vi "Message Console.vi"(7 "Name":string="MessageConsole") -> ()   [LabVIEW 2017, in "DebugConsole.lvlib"]
doc: "CSM Debug Console, you can use this tool:\n\n1. Select an existing CSM instance, open the front panel and block diagram.\n2. Scan the API interfaces of existing CSM instances.\n3. Select an API interface, call synchronously or asynchronously, view the return value.\n4. View the overall program's running log."
uses:
  DebugConsole.lvlib
  _Support/GlobalEvent/LogFilter/LogFilter.lvclass/LogFilter.ctl
  _Support/Typedef/_CSM_GlobalLog_MSG.ctl
  _Support/Typedef/_CSM_Response Source Message.ctl
  _Support/Typedef/_CSM_GlobalLog_MSG_TYPE.ctl
  _Support/Typedef/_CSM_List Module Scope.ctl
  _BroadcastDef.ctl
  _Polymophic/Build Synchronous Message with Arguments.vi
  _Polymophic/Build No-Reply Asynchronous Message with Arguments.vi
  _Polymophic/Build Interrupt Broadcast Message.vi
  AdvanceAPI/CSM - Convert Error to Argument.vi
  _Support/GlobalEvent/GEvt-Generate with Rule Check.vi
  _Support/GlobalEvent/Cache-GEvt Filter Object.vi
  _Support/GlobalEvent/Cache-GEvt Refs.vi
  AdvanceAPI/CSM - Keywords.vi
  _Shared/Trim Single-line Text.vi
  _Support/Message/Parse State with Arguments String.vi
  _Support/GlobalEvent/LogFilter/LogFilter - Check.vi
  _Support/GlobalEvent/GEvt-Convert Filter Rules - v1.2.vi
  _Support/ChangeFlag/FlagInstance-GEvt Filter.vi
  _Support/GlobalEvent/GEvt-Valid Subscribers.vi
  _Support/ChangeFlag/FlagInstance-GEvt Refs.vi
  _Support/GlobalEvent/LogFilter/CheckVIs/Group Check - LogType.vi
  _Support/GlobalEvent/LogFilter/CheckVIs/Group Check - CSM.vi
  _Support/GlobalEvent/LogFilter/CheckVIs/Group Check - State.vi
  _Support/GlobalEvent/LogFilter/CheckVIs/CSM Check - LogType.vi
  _Support/GlobalEvent/LogFilter/CheckVIs/CSM Check - State.vi
  _Support/GlobalEvent/LogFilter/CheckVIs/CSM Check - StateType.vi
  _Support/GlobalEvent/LogFilter/CheckVIs/Group Check - StateType.vi
  _Support/GlobalEvent/LogFilter/CheckVIs/CSM Check - Broadcast.vi
  _Support/GlobalEvent/LogFilter/CheckVIs/Group Check - Broadcast.vi
  _Support/GlobalEvent/LogFilter/CheckVIs/Group Check - UserLog.vi
  _Support/GlobalEvent/LogFilter/CheckVIs/CSM Check - UserLog.vi
  _Support/GlobalEvent/LogFilter/SettingVIs/Set Global CSM Filter.vi
  _Support/GlobalEvent/LogFilter/SettingVIs/Set Global LogType Filter.vi
  _Support/GlobalEvent/LogFilter/SettingVIs/Set Global State Filter.vi
  _Support/GlobalEvent/LogFilter/SettingVIs/Set CSM LogType Filter.vi
  _Support/GlobalEvent/LogFilter/SettingVIs/Set CSM State Filter.vi
  _Support/GlobalEvent/LogFilter/SettingVIs/Set Global StateType Filter.vi
  _Support/GlobalEvent/LogFilter/SettingVIs/Set CSM StateType Filter.vi
  _Support/GlobalEvent/LogFilter/SettingVIs/Set Periodic Log Filter.vi
  _Support/GlobalEvent/LogFilter/SettingVIs/Set CSM Broadcast Filter.vi
  _Support/GlobalEvent/LogFilter/SettingVIs/Set Global Broadcast Filter.vi
  _Support/GlobalEvent/LogFilter/SettingVIs/Set Global UserLog Filter.vi
  _Support/GlobalEvent/LogFilter/SettingVIs/Set CSM UserLog Filter.vi
  _Support/ChangeFlag/ChangeFlag-Read.vi
  _Support/GlobalEvent/LogFilter/Support/Log State Type.vi
  _csmlite/_PassAllowedMessage - MsgList.vi
  _Support/ChangeFlag/ChangeFlagDB.vi
  _Support/GlobalEvent/FGV-GlobalEventRef(lvlibp).vi
  _Support/GlobalEvent/FGV-GlobalEventQueues(lvlibp).vi
  _Support/GlobalEvent/FGV-GEvt Filter Rules(lvlibp).vi
  _Support/GlobalEvent/LogFilter/LogFilter.lvclass
  Communicable State Machine.lvlib
  _Shared/CSM Shared.lvlib
  _ui/csm-ui-support.lvlib
  _csmlite/_csmlite.lvlib
  <vilib>/UserTags/UserTags.lvlib
  _csmHelper/API with lvcsm Support/CSM-Helper API with lvcsm Support.lvlib
panel:
  in  "CSM":string
  in  "Timeout(s)":i32=10 caption="(s)" min=1 max=180 step=1 format="%.0p"
  in  "Interface-Filter":enum16{"API-Only", "UserDef States", "All"}(ring)
  in  "Refresh API":bool
  in  "MsgString":string(combo)
  in  "Sync (-@)":bool
  in  "Async (->|)":bool
  in  "Arguments":string
  in  "Revert Safe String":bool=TRUE
  out "Response":string
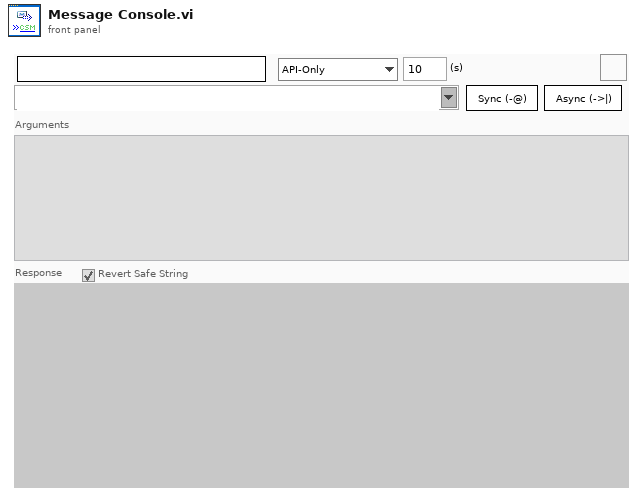
[diagram p1: front panel]
types:
  T1 = enum32{"Invalid", "Standard", "Closed", "Hidden", "Minimized", "Maximized"}
  T2 = enum32{"invalid app kind", "Development System", "Run Time System", "Student Edition", "Embedded LabVIEW", "Evaluation", "Custom"}
  T3 = typedef "Communicable State Machine.lvlib/_CSM_List Module Scope.ctl" = enum16{"Normal", "System Only", "All"}
  T4 = typedef "DebugConsole.lvlib/_BroadcastDef.ctl" = enum16{"<no action>", "Macro: Exit", "CSM: Module List Changed", "CSM: Scripts Changed", "CSM: Registration Changed", "CSM: Module Selected", "CSM: Message Excuted", "CSM: Broadcast Excuted", "CSM: Registration Action Excuted", "UI: Try to Change Command"}
  T5 = cluster{"Shift":bool, "Ctrl":bool, "Alt":bool, "Cmd":bool, "Opt":bool}
  T6 = cluster{"Core":cluster{"Current VI Reference":refnum<vi>, "Close Panel on Exit?":bool}, "CSM Global Log Event":refnum<user-event>, "Toobar.advance":refnum<vi>[], "CSM Check History":string[], "History Length":i32}
  T7 = cluster{"Current VI Reference":refnum<vi>, "Close Panel on Exit?":bool}
  T8 = enum8{"Enabled", "Disabled", "Disabled and Grayed Out"}
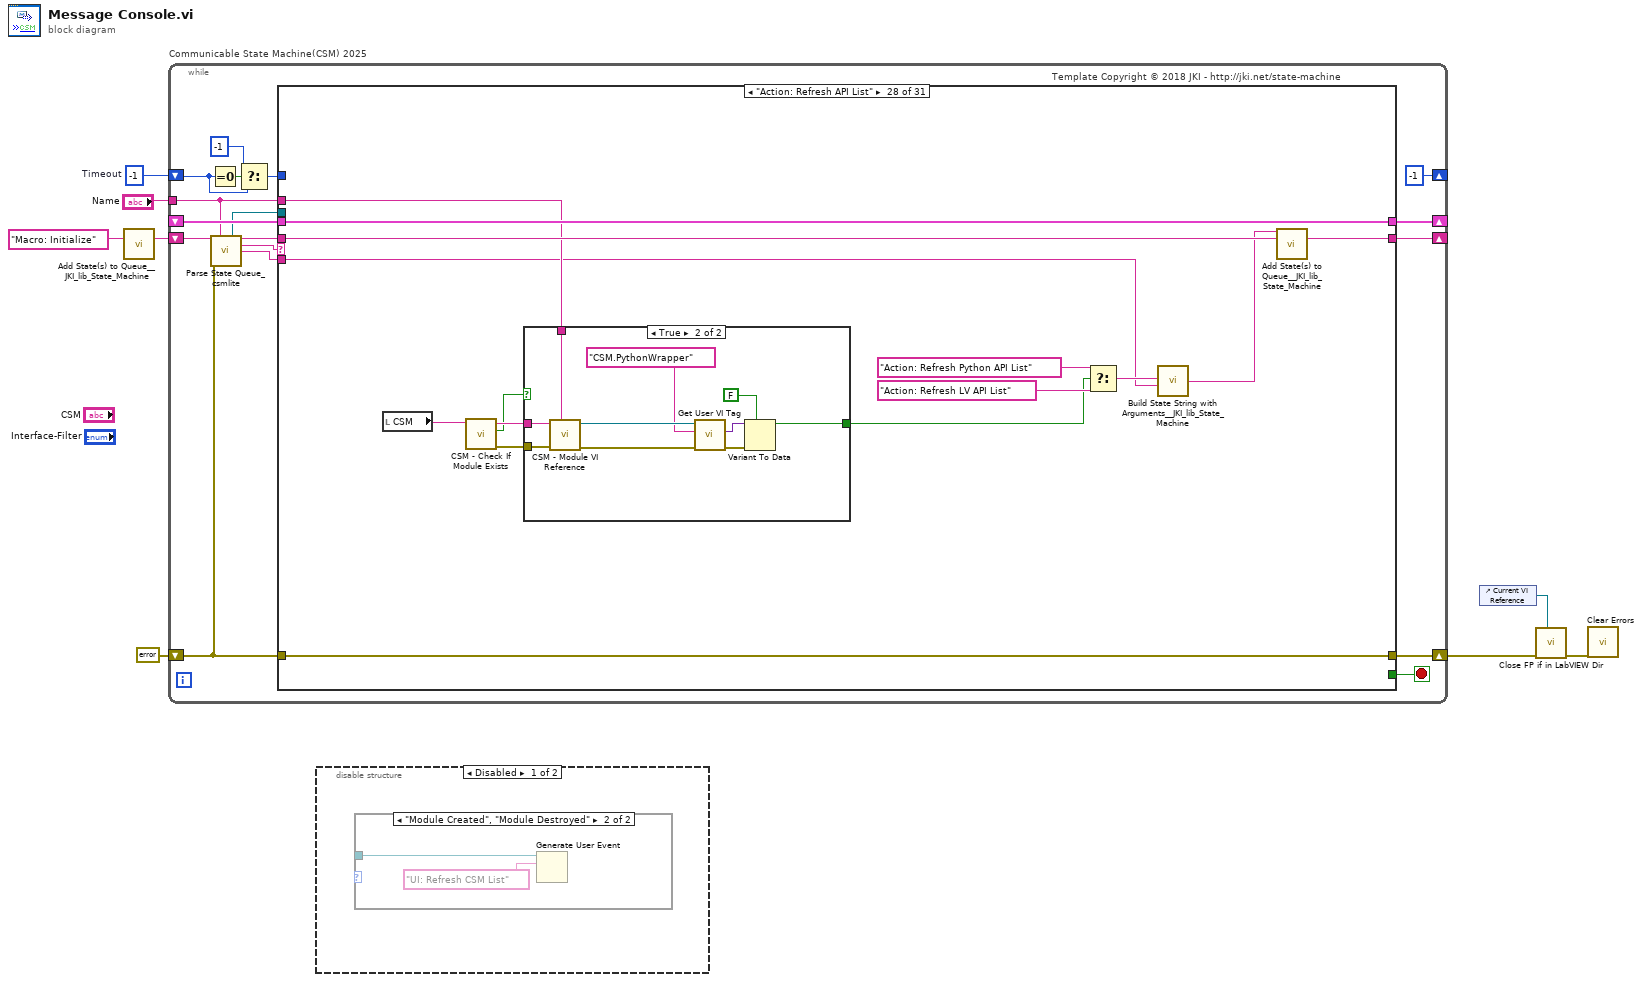
[diagram p0: block diagram]
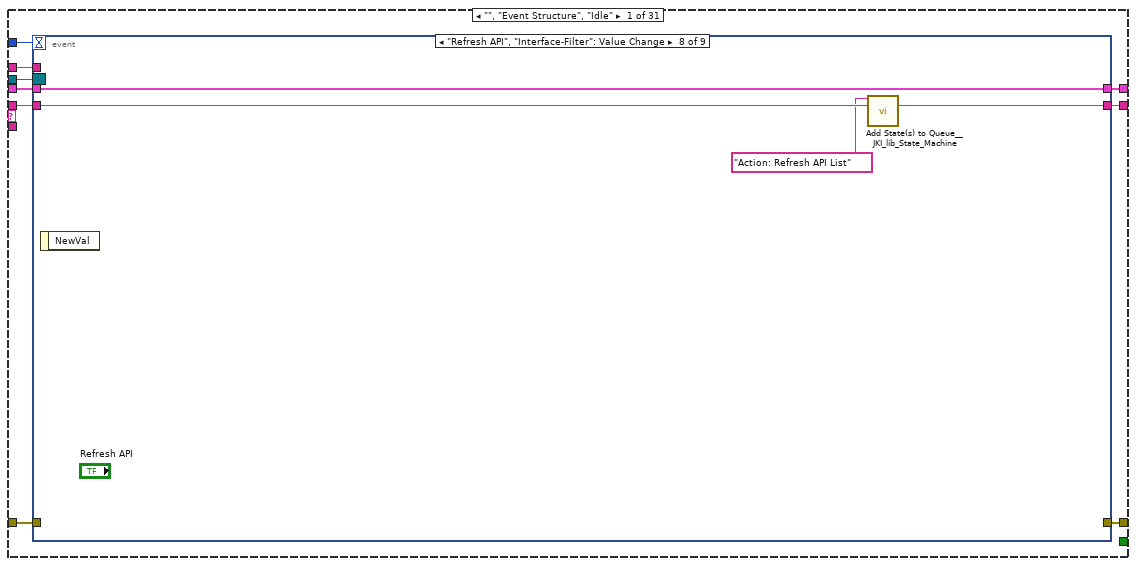
[diagram p4: hidden frame]
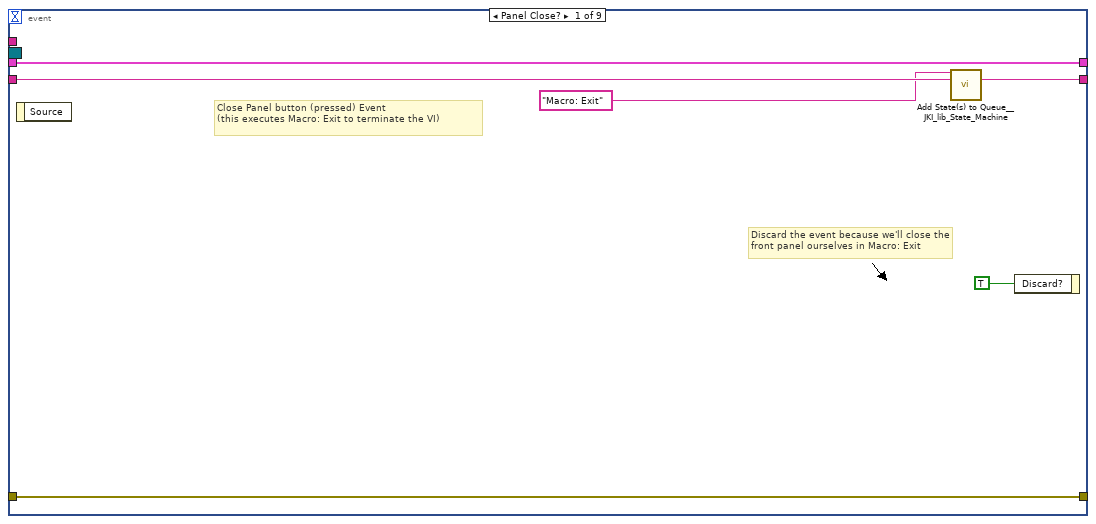
[diagram p5: hidden frame]
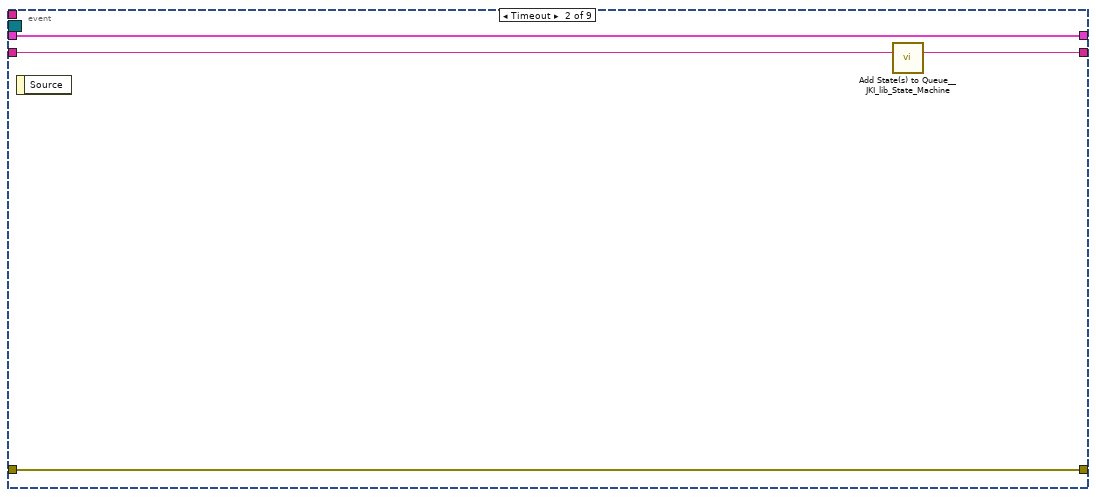
[diagram p6: hidden frame]
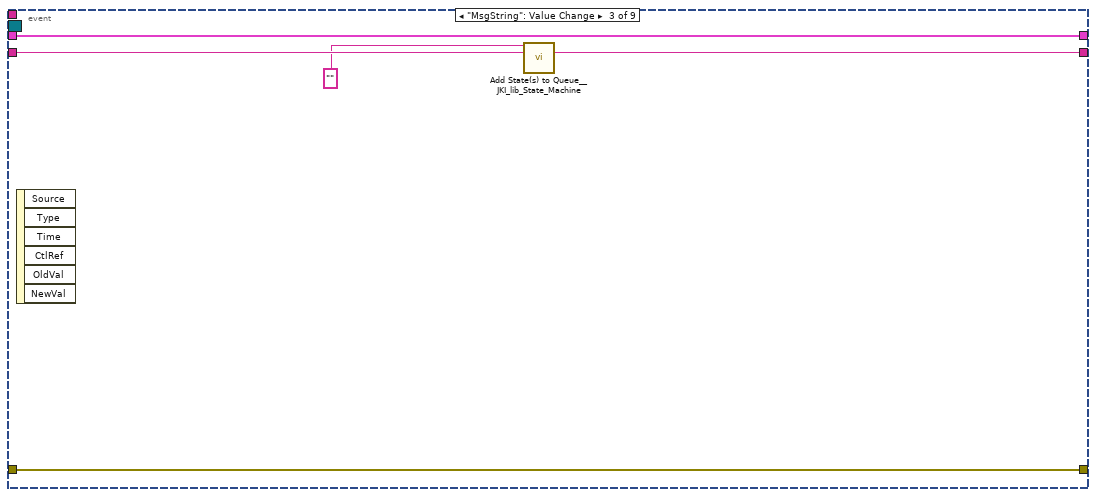
[diagram p7: hidden frame]
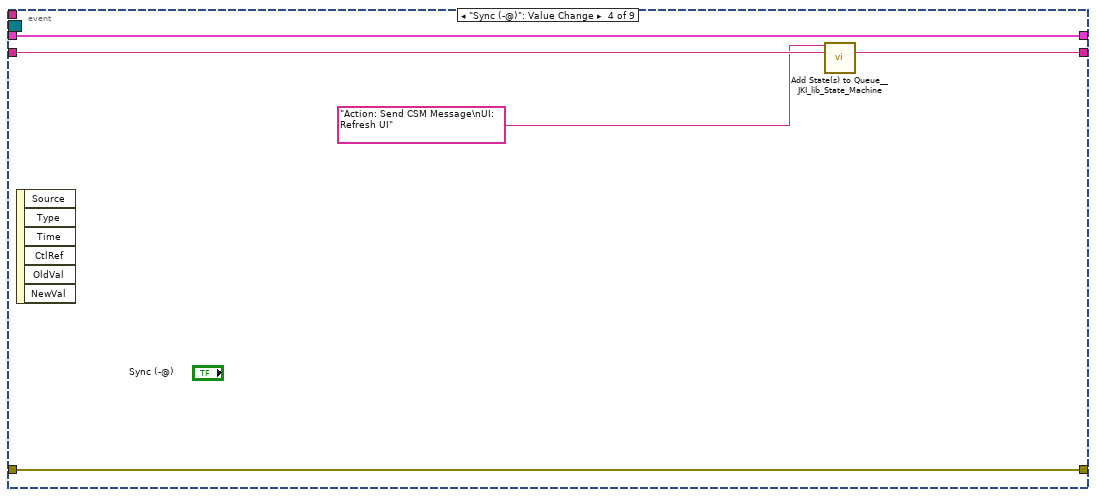
[diagram p8: hidden frame]
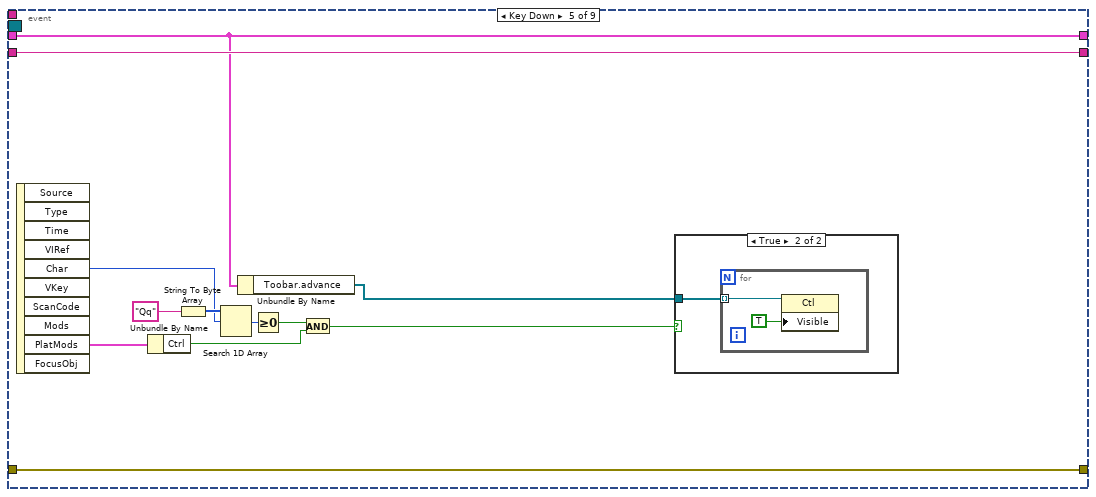
[diagram p9: hidden frame]
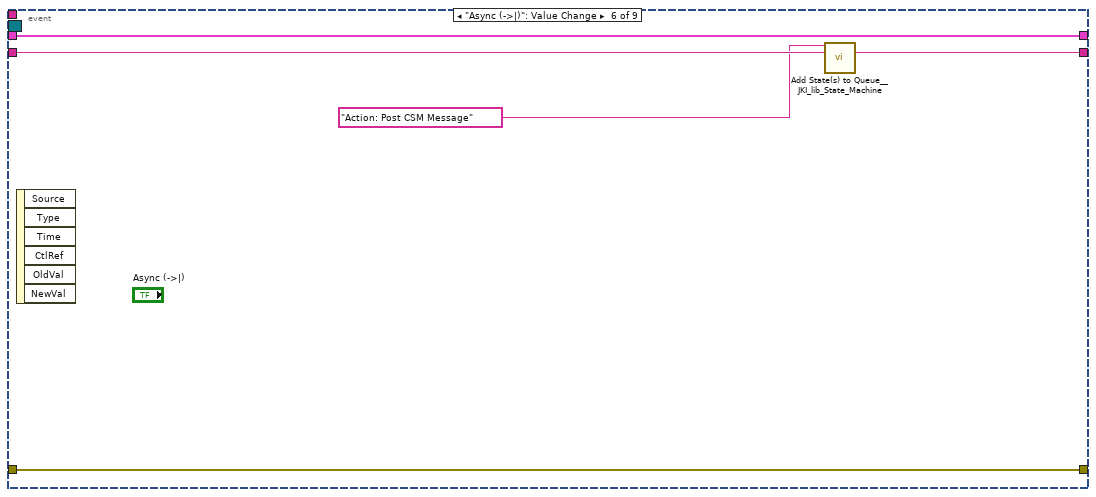
[diagram p11: hidden frame]
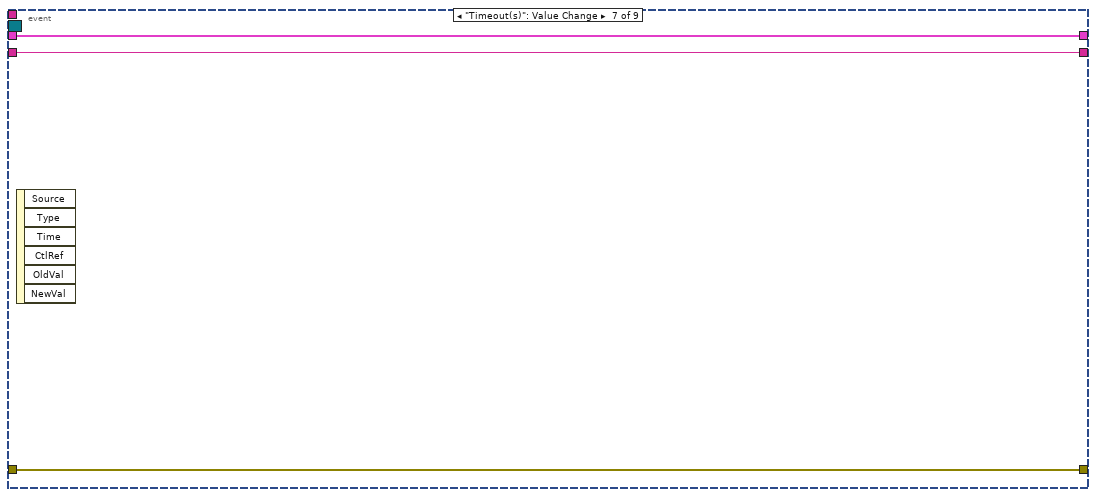
[diagram p12: hidden frame]
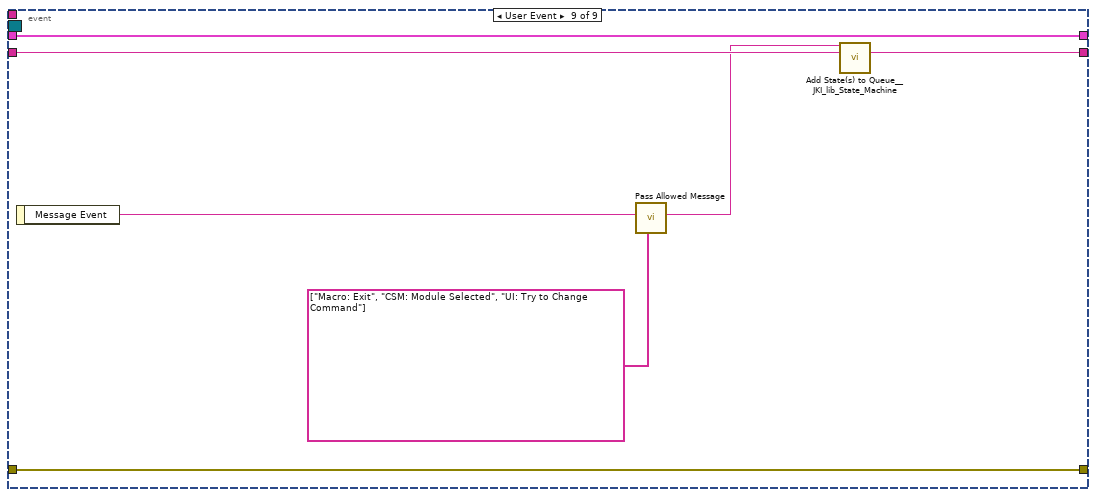
[diagram p13: hidden frame]
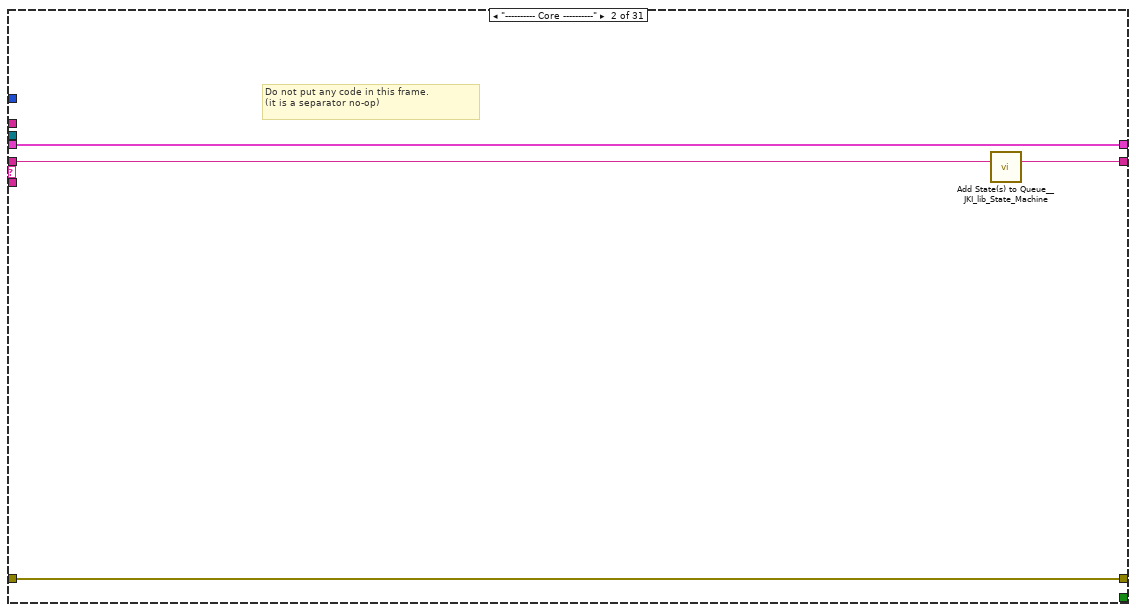
[diagram p14: hidden frame]
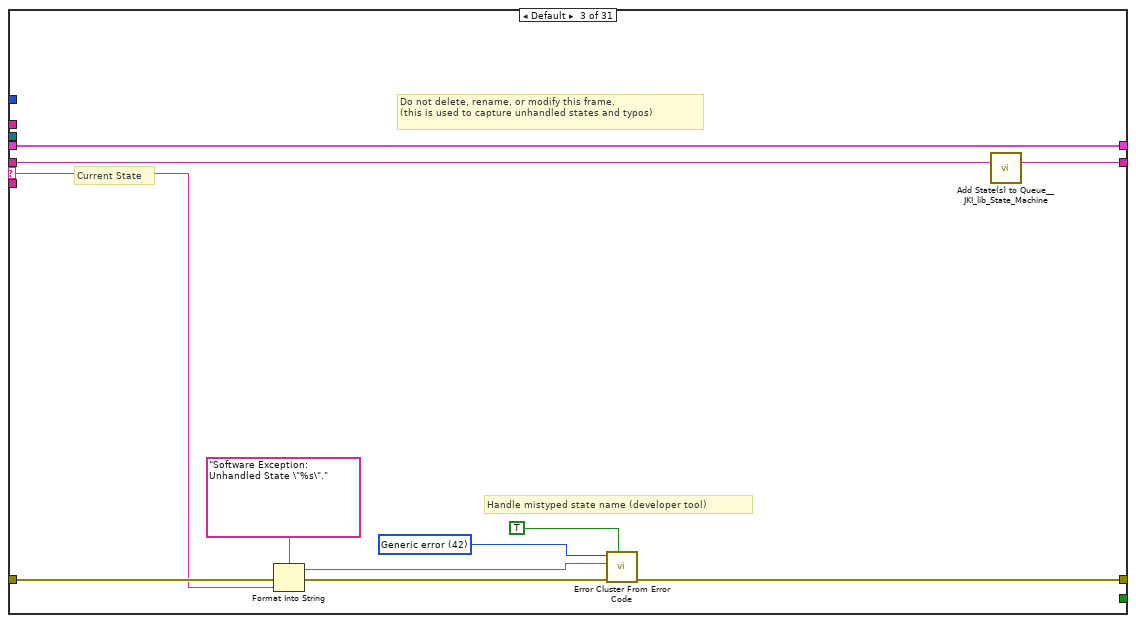
[diagram p15: hidden frame]
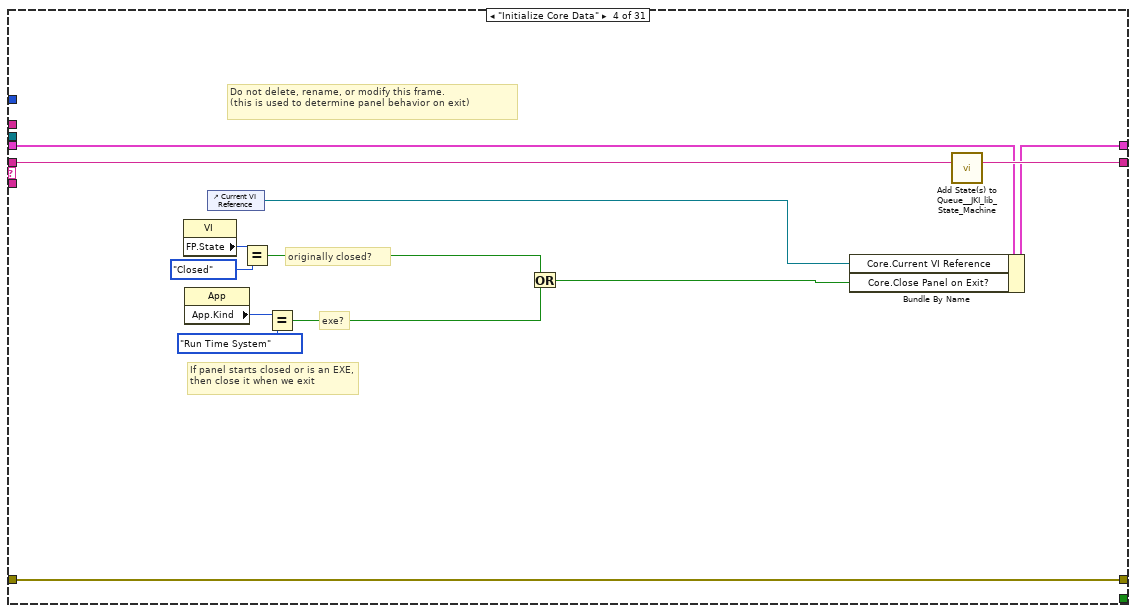
[diagram p16: hidden frame]
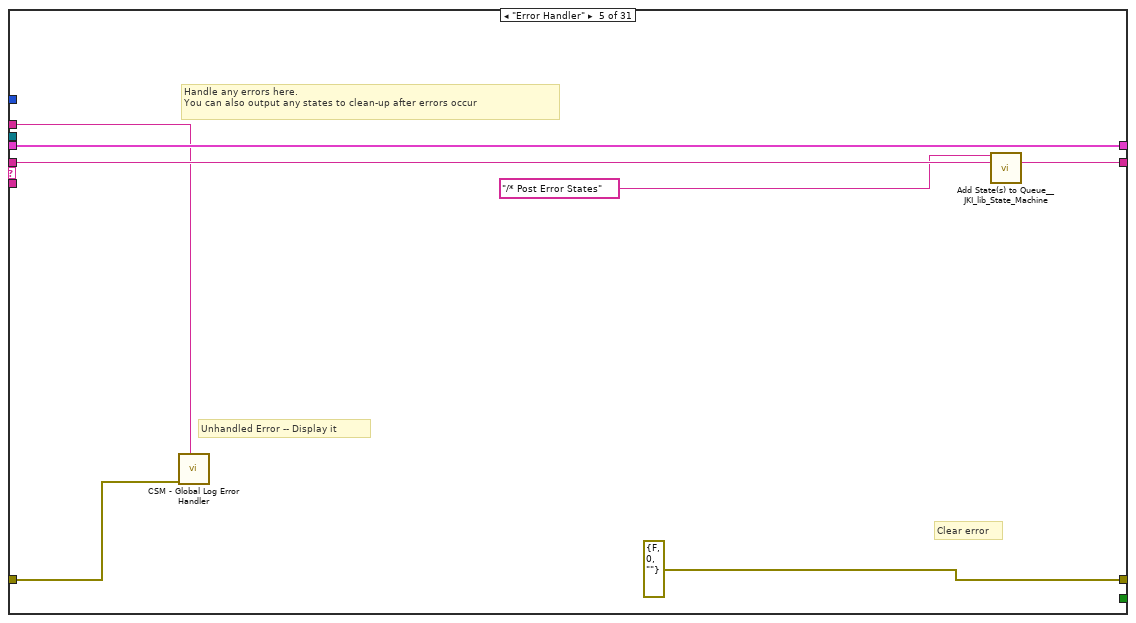
[diagram p17: hidden frame]
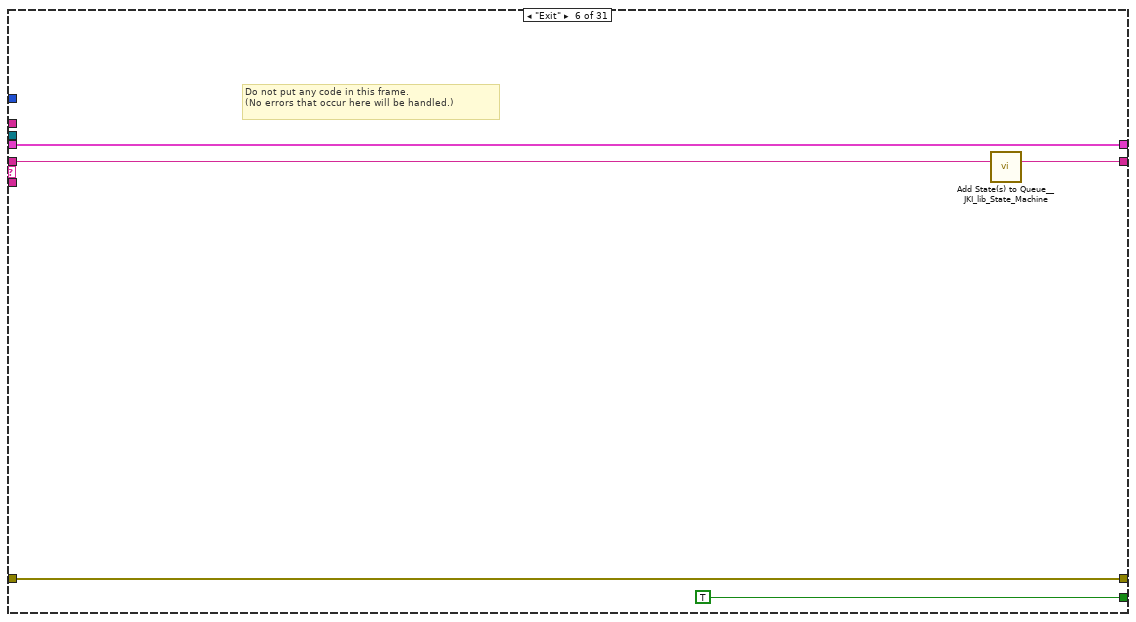
[diagram p18: hidden frame]
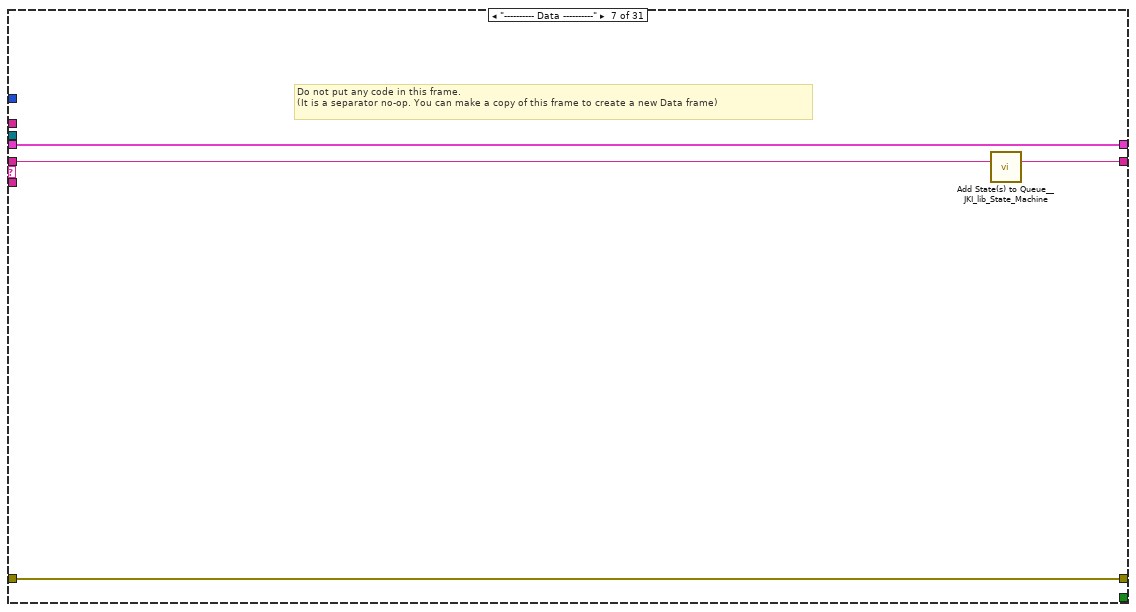
[diagram p19: hidden frame]
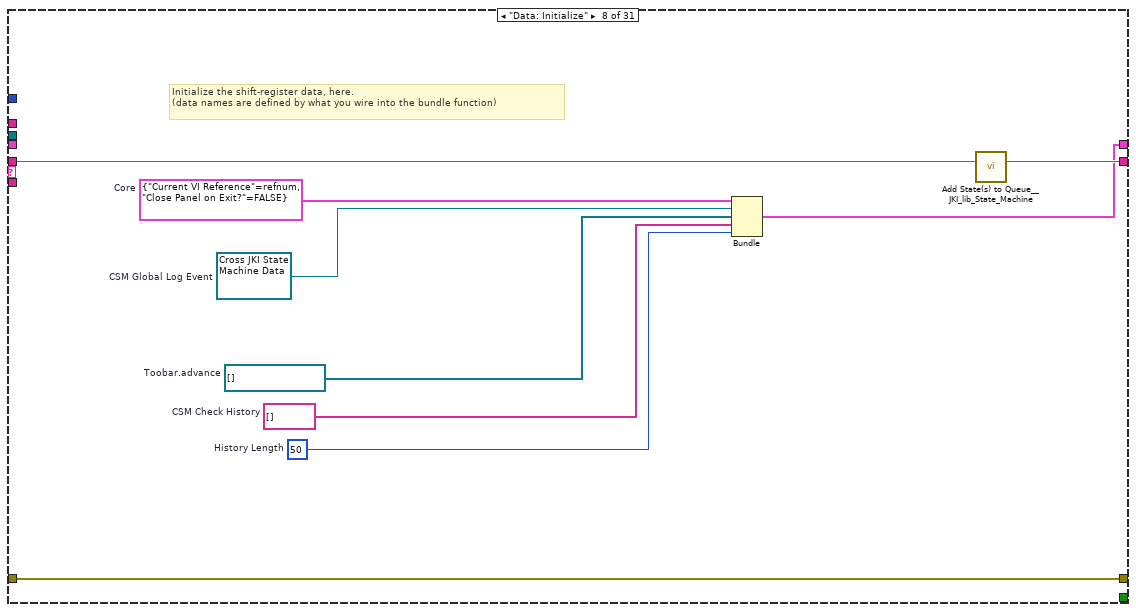
[diagram p20: hidden frame]
diagram:
  w6 = -1  # Timeout
  n1 = call <vilib>:"Add State(s) to Queue__JKI_lib_State_Machine.vi"("State(s) in (\"\")"="Macro: Initialize") -> ("States Out"=w7:string)  [unwired: 14 in]
  n2 = while "Communicable State Machine(CSM) 2025" {
    shift-right: [w18] -> _
    shift-left: _ -> [w17]
    shift-right: [w21] -> w3
    shift-left: errorcluster {"status"=FALSE, "code"=0, "source"=""} ("error out") -> [w16]
    shift-right: [w20] -> _
    shift-left: w7 -> [w22]
    tunnel: "Name" -> [w10]
    shift-right: [-1 ("Timeout")] -> _
    shift-left: w6 -> [w13]
    stop <- w19 stop-if-true
    # "Template Copyright © 2018 JKI - http://jki.net/state-machine"
    n3 = Equal To 0?(x=w13) -> (x = 0?=w15:bool)
    n4 = call "Parse State Queue_csmlite.vi"("State Queue"=w22, "Current Module(\"\" to generate an ID)"=w10, "Error In (no error)"=w16) -> ("Event Registration Refnum"=w9:refnum<event-registration>, "Remaining States"=w24:string, "Current State"=w25:string, "Arguments"=w23:string)  [unwired: 9 in]
    n5 = Select(t=-1 ("Timeout"), s=w15, f=w13) -> (s? t:f=w12:i32)
    n6 = case shown="\"Action: Refresh API List\"" w25 {
      selector: w25 -> [_ _ w93 _ _ _ _ _ _ _ _ _ _ _ _ _ _ _ _ _ _ _ _ _ _ _ _ _ _ _ _]
      tunnel: w24 -> [w34 w92 w97 w116 w123 w128 w132 w141 w143 w150 w154 w161 w170 w181 w256 w263 w266 w272 w276 w302 w307 w314 w318 w328 w350 w366 w380 w393 w418 w448 w489]
      tunnel: w23 -> [_ _ _ _ _ _ _ _ _ _ _ _ w165 w175 w255 _ w268 _ w286 _ _ _ _ _ _ _ _ w382 w407 w437 _]
      tunnel: w17 -> [w32 w89 w95 w109 w120 w126 w129 _ w142 w145 w151 w158 w168 w177 w253 w262 w269 w271 w292 w299 w304 w311 w315 w326 w348 w364 w379 w395 w414 w444 w488]
      tunnel: [w31 w90 w99 w113 errorcluster {"status"=FALSE, "code"=0, "source"=""} ("error out") w125 w130 w138 w144 w146 w152 w159 w166 w178 w257 w264 w270 w273 w293 w300 w305 w312 w316 _ _ w363 w381 w396 _ _ w490] -> w21
      tunnel: w16 -> [w30 w90 w98 w113 w119 w125 w130 w138 w144 w147 w152 w159 w167 w179 w257 w264 w270 w273 w293 w300 w305 w312 w316 _ _ _ w381 w396 _ _ w490]
      tunnel: [w33 w91 w96 w115 w122 w127 w131 w140 w143 w149 w153 w160 w169 w180 w256 w263 w267 w272 w277 w301 w306 w313 w317 w327 w349 w365 w380 w394 w418 w448 w489] -> w20
      tunnel: [_ _ _ _ _ TRUE _ _ _ _ _ _ _ _ _ _ _ _ _ _ _ _ _ _ _ _ _ _ _ _ _] -> w19
      tunnel: [w29 w89 w95 w114 w120 w126 w129 w139 w142 w145 w151 w158 w168 w177 w253 w262 w269 w271 w292 w299 w304 w311 w315 w326 w348 w364 w379 w395 w413 w443 w488] -> w18
      tunnel: w12 -> [w28 _ _ _ _ _ _ _ _ _ _ _ _ _ _ _ _ _ _ _ _ _ _ _ _ _ _ _ _ _ _]
      tunnel: w10 -> [w27 _ _ _ w117 _ _ _ _ _ _ _ _ _ _ _ _ _ _ _ _ _ _ _ _ _ _ w389 w416 w446 _]
      tunnel: w9 -> [w26 _ _ _ _ _ _ _ _ _ _ _ _ _ _ _ _ _ _ _ _ _ _ _ _ _ _ _ _ _ _]
      frame "", "Event Structure", "Idle" {
        n7 = event shown="[7] \"Refresh API\", \"Interface-Filter\": Value Change" {
          selector: w26 -> [_ _ _ _ _ _ _ _ _]
          dyn-events: _ -> [_ _ _ _ _ _ _ _ _]
          timeout: w28 -> [_ _ _ _ _ _ _ _ _]
          tunnel: w34 -> [w40 w44 w46 w51 w66 w71 w77 w79 w85]
          tunnel: [w39 w43 w47 w52 w66 w72 w77 w80 w86] -> w33
          tunnel: w32 -> [w37 w41 w48 w53 w55 w73 w75 w81 w87]
          tunnel: [w38 w42 w49 w54 w65 w74 w76 _ w88] -> w31
          tunnel: w30 -> [w38 w42 w49 w54 w65 w74 w76 _ w88]
          tunnel: [w37 w41 w48 w53 w55 w73 w75 w81 w87] -> w29
          tunnel: w27 -> [_ _ _ _ _ _ _ _ _]
          event Panel Close? {
            # "Discard the event because we'll close the front panel ourselves in Macro: Exit"
            # "Close Panel button (pressed) Event\n(this executes Macro: Exit to terminate the VI)"
            n8 = event-data() -> ()  [unwired: 1 in, 1 out]
            n9 = call <vilib>:"Add State(s) to Queue__JKI_lib_State_Machine.vi"("State(s) in Front (\"\")"="Macro: Exit", "State(s) in (\"\")"=w40) -> ("States Out"=w39:string)  [unwired: 13 in]
            n10 = event-data("Discard?"=TRUE) -> ()  [unwired: 1 in, 1 out]
          }
          event Timeout {
            n11 = event-data() -> ()  [unwired: 1 in, 1 out]
            n12 = call <vilib>:"Add State(s) to Queue__JKI_lib_State_Machine.vi"("State(s) in (\"\")"=w44) -> ("States Out"=w43:string)  [unwired: 14 in]
          }
          event "MsgString": Value Change {
            n13 = event-data() -> ()  [unwired: 1 in, 6 out]
            n14 = call <vilib>:"Add State(s) to Queue__JKI_lib_State_Machine.vi"("State(s) in Front (\"\")"="" ("State(s) in Front (\"\")"), "State(s) in (\"\")"=w46) -> ("States Out"=w47:string)  [unwired: 13 in]
          }
          event "Sync (-@)": Value Change {
            n15 = event-data() -> ()  [unwired: 1 in, 6 out]
            n16 = call <vilib>:"Add State(s) to Queue__JKI_lib_State_Machine.vi"("State(s) in Front (\"\")"="Action: Send CSM Message\nUI: Refresh UI" ("State(s) in Front (\"\")"), "State(s) in (\"\")"=w51) -> ("States Out"=w52:string)  [unwired: 13 in]
          }
          event Key Down {
            n17 = event-data() -> ("Char"=w56:i16, "PlatMods"=w57:T5)  [unwired: 1 in, 8 out]
            n18 = Unbundle By Name(w57) -> ("Ctrl"=w60:bool)
            n19 = String To Byte Array(string="Qq") -> (unsigned byte array=w62:u8[])
            n20 = Search 1D Array(1D array=w62, element=w56) -> (index of element=w63:i32)  [unwired: 1 in]
            n21 = Unbundle By Name(w55) -> ("Toobar.advance"=w58:refnum<vi>[])
            n22 = Greater Or Equal To 0?(x=w63) -> (x >= 0?=w64:bool)
            n23 = And(x=w64, y=w60) -> (x .and. y?=w59:bool)
            n24 = case shown="True" w59 {
              tunnel: w58 -> [_ w67]
              frame False {
              }
              frame True {
                n25 = for {
                  tunnel: w67 -> [w69] mode=indexing
                  n26 = property class="Ctl"(reference=w69, "Visible"=TRUE) -> ()  [unwired: 1 in, 2 out]
                }
              }
            }
          }
          event "Async (->|)": Value Change {
            n27 = event-data() -> ()  [unwired: 1 in, 6 out]
            n28 = call <vilib>:"Add State(s) to Queue__JKI_lib_State_Machine.vi"("State(s) in Front (\"\")"="Action: Post CSM Message" ("State(s) in Front (\"\")"), "State(s) in (\"\")"=w71) -> ("States Out"=w72:string)  [unwired: 13 in]
          }
          event "Timeout(s)": Value Change {
            n29 = event-data() -> ()  [unwired: 1 in, 6 out]
          }
          event "Refresh API", "Interface-Filter": Value Change {
            n30 = event-data() -> ()  [unwired: 1 in, 1 out]
            n31 = call <vilib>:"Add State(s) to Queue__JKI_lib_State_Machine.vi"("State(s) in Front (\"\")"="Action: Refresh API List" ("State(s) in Front (\"\")"), "State(s) in (\"\")"=w79) -> ("States Out"=w80:string)  [unwired: 13 in]
          }
          event User Event {
            n32 = event-data() -> ("Message Event"=w84:string)  [unwired: 1 in]
            n33 = call-poly "Pass Allowed Message.vi"("Allowed Message"=string[] ["Macro: Exit", "CSM: Module Selected", "UI: Try to Change Command"], "JKISM External Event"=w84) -> ("States"=w83:string)  [unwired: 7 in]
            n34 = call <vilib>:"Add State(s) to Queue__JKI_lib_State_Machine.vi"("State(s) in Front (\"\")"=w83, "State(s) in (\"\")"=w85) -> ("States Out"=w86:string)  [unwired: 13 in]
          }
        }
      }
      frame "---------- Core ----------" {
        # "Do not put any code in this frame.\n(it is a separator no-op)"
        n35 = call <vilib>:"Add State(s) to Queue__JKI_lib_State_Machine.vi"("State(s) in (\"\")"=w92) -> ("States Out"=w91:string)  [unwired: 14 in]
      }
      frame Default {
        w102 = 42 items=["No error", "Argument error", "Memory is full", "Out of zone", "End of file", "File already open", "Generic file I/O error", "File not found", "File permission error", "Disk is full", "Duplicate path", "Too many files open", "System feature not enabled", "Resource file not found", "Cannot add resource", "Resource not found", "Image not found", "Image memory error", "Pen does not exist", "Config type invalid", "Config token not found", "Config parse error", "Config memory error", "Bad external code format", "Bad external code offset", "External code not present", "Null window", "Destroy window error", "Null menu", "Print aborted", "Bad print record", "Print driver error", "Windows error during printing", "Memory error during printing", "Print dialog error", "Generic print error", "Invalid device refnum", "Device not found", "Device parameter error", "Device unit error", "Cannot open device", "Device call aborted", "Generic error", "Cancelled by user", "Object ID too low", "Object ID too high", "Object not in heap", "Unknown heap", "Unknown object (invalid DefProc)", "Unknown object (DefProc not in table)", "Message out of range", "Invalid (null) method", "Unknown message", "Manager call not supported", "Bad address", "Network operation in progress", "Network operation timed out", "Connection is busy", "Network attribute not supported", "Network error", "Address in use", "System out of memory", "Connection aborted", "Connection refused", "Not connected", "Already connected", "Connection closed", "Initialization error (interapplication manager)", "Bad occurrence", "Wait on unbound occurrence handler", "Occurrence queue overflow", "Datalog type conflict", "Unused", "Unrecognized type (interapplication manager)", "Memory corrupt", "Failed to make temporary DLL", "Old CIN version", "Drag socket not found", "Failed to load drop-object", "Failed to register OLE object", "Failed to release OLE object", "Format specifier type mismatch", "Unknown format specifier", "Too few format specifiers", "Too many format specifiers", "Scan failed", "Newer CIN version", "Error converting to variant", "Runtime menu error", "Password tampered", "Variant attribute not found", "Incompatible variant data type", "Event data is not available", "Event Store is not present", "Occurrence is not found", "Event Queue is not created", "Event info is not available", "Refnum passed is NULL", "Error retrieving Class GUID", "Error retrieving CoClass GUID", "Error retrieving TypeLib GUID.", "Bad built application magic bytes.", "Specific driver is different from the specific driver associated with the Logical Name.", "There is no session opened to the class driver.", "Max Error", "MAX - Error with config objects", "MAX - Error loading configuration", "MAX - Group not supported"]
        # "Current State"
        # "Do not delete, rename, or modify this frame.\n(this is used to capture unhandled states and typos)"
        # "Handle mistyped state name (developer tool)"
        n36 = Format Into String(format string="Software Exception: Unhandled State \"%s\"." ("message"), error in=w98, w93) -> (resulting string=w101:string, error out=w100:errorcluster)  [unwired: 1 in]
        n37 = call <vilib>:"Error Cluster From Error Code.vi"("show call chain? (False)"=TRUE, "error in (no error)"=w100, "error message (\"\")"=w101, "error code (0)"=w102) -> ("error out"=w99:errorcluster)  [unwired: 5 in]
        n38 = call <vilib>:"Add State(s) to Queue__JKI_lib_State_Machine.vi"("State(s) in (\"\")"=w97) -> ("States Out"=w96:string)  [unwired: 14 in]
      }
      frame "Initialize Core Data" {
        # "Do not delete, rename, or modify this frame.\n(this is used to determine panel behavior on exit)"
        # "originally closed?"
        # "exe?"
        # "If panel starts closed or is an EXE, then close it when we exit"
        n39 = property class="VI"() -> ("FP.State"=w106:T1)  [unwired: 2 in, 2 out]
        n40 = property class="App"() -> ("App.Kind"=w112:T2)  [unwired: 2 in, 2 out]
        n41 = control-ref of="Current VI Reference"() -> (w107:refnum<vi>)
        n42 = Equal?(x=w106, y=T1."Closed" ("Front Panel Window:State")) -> (x = y?=w104:bool)
        n43 = Equal?(x=w112, y=T2."Run Time System" ("Application:Kind")) -> (x = y?=w110:bool)
        n44 = Or(x=w104, y=w110) -> (x .or. y?=w108:bool)
        n45 = Bundle By Name(cluster=w109, "Core.Current VI Reference"=w107, "Core.Close Panel on Exit?"=w108) -> (w114:T6)
        n46 = call <vilib>:"Add State(s) to Queue__JKI_lib_State_Machine.vi"("State(s) in (\"\")"=w116) -> ("States Out"=w115:string)  [unwired: 14 in]
      }
      frame "Error Handler" {
        # "Unhandled Error -- Display it"
        # "Handle any errors here.\nYou can also output any states to clean-up after errors occur"
        # "Clear error"
        n47 = call "CSM - Global Log Error Handler.vi"("Place (\"\" to Use VI's Name)"=w117, "Error In"=w119) -> ()  [unwired: 9 in, 1 out]
        n48 = call <vilib>:"Add State(s) to Queue__JKI_lib_State_Machine.vi"("State(s) in Front (\"\")"="/* Post Error States", "State(s) in (\"\")"=w123) -> ("States Out"=w122:string)  [unwired: 13 in]
      }
      frame "Exit" {
        # "Do not put any code in this frame.\n(No errors that occur here will be handled.)"
        n49 = call <vilib>:"Add State(s) to Queue__JKI_lib_State_Machine.vi"("State(s) in (\"\")"=w128) -> ("States Out"=w127:string)  [unwired: 14 in]
      }
      frame "---------- Data ----------" {
        # "Do not put any code in this frame.\n(It is a separator no-op. You can make a copy of this frame to create a new Data frame)"
        n50 = call <vilib>:"Add State(s) to Queue__JKI_lib_State_Machine.vi"("State(s) in (\"\")"=w132) -> ("States Out"=w131:string)  [unwired: 14 in]
      }
      frame "Data: Initialize" {
        w133 = 50  # History Length
        w134 = string[] []  # CSM Check History
        w135 = refnum<vi>[] []  # Toobar.advance
        w136 = refnum<user-event> refnum  # CSM Global Log Event
        w137 = T7 {"Current VI Reference"=refnum, "Close Panel on Exit?"=FALSE}  # Core
        # "Initialize the shift-register data, here.\n(data names are defined by what you wire into the bundle function)"
        n51 = Bundle("Core"=w137, "CSM Global Log Event"=w136, "Toobar.advance"=w135, "CSM Check History"=w134, "History Length"=w133) -> (w139:T6)  [unwired: 1 in]
        n52 = call <vilib>:"Add State(s) to Queue__JKI_lib_State_Machine.vi"("State(s) in (\"\")"=w141) -> ("States Out"=w140:string)  [unwired: 14 in]
      }
      frame "Data: Initialize References" {
      }
      frame "Data: Cleanup" {
        # "Cleanup any data and references, here.\n(this is called automatically, by the Macro: Exit)"
        n53 = Unbundle By Name(w145) -> ("Core.Current VI Reference"=w148:refnum<vi>)
        n54 = Close Reference(reference=w148, error in (no error)=w147) -> (error out=w146:errorcluster)
        n55 = call <vilib>:"Add State(s) to Queue__JKI_lib_State_Machine.vi"("State(s) in (\"\")"=w150) -> ("States Out"=w149:string)  [unwired: 14 in]
      }
      frame "---------- UI ----------" {
        # "Do not put any code in this frame.\n(It is a separator no-op. You can make a copy of this frame to create a new UI frame)"
        n56 = call <vilib>:"Add State(s) to Queue__JKI_lib_State_Machine.vi"("State(s) in (\"\")"=w154) -> ("States Out"=w153:string)  [unwired: 14 in]
      }
      frame "UI: Initialize" {
        # "Initialize the User Interface, here.\n(this is called automatically, by the Macro: Init)"
        n57 = Unbundle By Name(w158) -> ("Toobar.advance"=w157:refnum<vi>[])
        n58 = disable-structure shown="Disabled" {
          disable-tunnel: w157 -> [w162 _]
          frame Disabled {
            n59 = for {
              tunnel: w162 -> [w164] mode=indexing
              n60 = property class="Ctl"(reference=w164, "Visible"=FALSE) -> ()  [unwired: 1 in, 2 out]
            }
          }
          frame Enabled {
          }
        }
        n61 = local write "Response"(" " ("State History")) -> ()
        n62 = local write "Interface-Filter"(enum16{"API-Only", "UserDef States", "All"}."UserDef States" ("Interface-Filter")) -> ()
        n63 = call <vilib>:"Add State(s) to Queue__JKI_lib_State_Machine.vi"("State(s) in (\"\")"=w161) -> ("States Out"=w160:string)  [unwired: 14 in]
      }
      frame "UI: Cursor Set" {
        # "Argument"
        # "Set and Unset Cursor Busy.\n(Usage: \"UI: Cursor Set >> Busy|Idle\")"
        n64 = case shown="\"Idle\", Default" w165 {
          tunnel: w167 -> [w172 w174]
          tunnel: [w171 w173] -> w166
          frame "Idle", Default {
            n65 = call <vilib>:"Unset Busy.vi"("error in (no error)"=w172) -> ("error out"=w171:errorcluster)  [unwired: 10 in]
          }
          frame "Busy" {
            n66 = call <vilib>:"Set Busy.vi"("error in (no error)"=w174) -> ("error out"=w173:errorcluster)  [unwired: 9 in, 1 out]
          }
        }
        n67 = call <vilib>:"Add State(s) to Queue__JKI_lib_State_Machine.vi"("State(s) in (\"\")"=w170) -> ("States Out"=w169:string)  [unwired: 14 in]
      }
      frame "UI: Front Panel State" {
        # "Argument"
        # "Set Front Panel Open or Closed\n(Usage: \"UI: Front Panel State >> Open|Close\")"
        n68 = Unbundle By Name(w177) -> ("Core.Current VI Reference"=w176:refnum<vi>)
        n69 = case shown="\"Minimize\", \"Minimized\"" w175 {
          tunnel: w179 -> [w187 w202 w213 w226 w239]
          tunnel: [w189 w203 w215 w228 w241] -> w178
          tunnel: w176 -> [w188 w200 w214 w227 w240]
          frame "Open", "Standard", Default {
            w182 = T1."Standard" ("State")
            n70 = property class="VI"(reference=w188, error in=w187) -> (reference out=w185:refnum<vi>, error out=w186:errorcluster, "FP.State"=w184:T1)
            n71 = Not Equal?(x=w184, y=w182) -> (x != y?=w183:bool)
            n72 = case shown="True" w183 {
              tunnel: [w193 w195] -> w189
              tunnel: w186 -> [w192 w195]
              tunnel: w185 -> [w191 _]
              tunnel: w182 -> [w190 _]
              frame True {
                n73 = invoke class="VI" method="FP.Open"(reference=w191, error in=w192, "Activate"=TRUE, "State"=w190) -> (error out=w193:errorcluster)  [unwired: 1 in, 4 out]
              }
              frame False {
              }
            }
          }
          frame "Close", "Closed" {
            n74 = property class="VI"(reference=w200, error in=w202) -> (reference out=w199:refnum<vi>, error out=w201:errorcluster, "FP.State"=w197:T1)
            n75 = Not Equal?(x=w197, y=T1."Closed" ("Front Panel Window:State")) -> (x != y?=w196:bool)
            n76 = case shown="True" w196 {
              tunnel: [w204 w207] -> w203
              tunnel: w201 -> [w204 w206]
              tunnel: w199 -> [_ w205]
              frame False {
              }
              frame True {
                n77 = invoke class="VI" method="FP.Close"(reference=w205, error in=w206) -> (error out=w207:errorcluster)  [unwired: 1 in, 2 out]
              }
            }
          }
          frame "Hidden", "Hide" {
            w208 = T1."Hidden" ("State")
            n78 = property class="VI"(reference=w214, error in=w213) -> (reference out=w211:refnum<vi>, error out=w212:errorcluster, "FP.State"=w210:T1)
            n79 = Not Equal?(x=w210, y=w208) -> (x != y?=w209:bool)
            n80 = case shown="True" w209 {
              tunnel: [w219 w220] -> w215
              tunnel: w212 -> [w218 w220]
              tunnel: w211 -> [w217 _]
              tunnel: w208 -> [w216 _]
              frame True {
                n81 = invoke class="VI" method="FP.Open"(reference=w217, error in=w218, "State"=w216) -> (error out=w219:errorcluster)  [unwired: 2 in, 4 out]
              }
              frame False {
              }
            }
          }
          frame "Minimize", "Minimized" {
            w221 = T1."Minimized" ("State")
            n82 = property class="VI"(reference=w227, error in=w226) -> (reference out=w224:refnum<vi>, error out=w225:errorcluster, "FP.State"=w223:T1)
            n83 = Not Equal?(x=w223, y=w221) -> (x != y?=w222:bool)
            n84 = case shown="True" w222 {
              tunnel: [w232 w233] -> w228
              tunnel: w225 -> [w231 w233]
              tunnel: w224 -> [w230 _]
              tunnel: w221 -> [w229 _]
              frame True {
                n85 = invoke class="VI" method="FP.Open"(reference=w230, error in=w231, "State"=w229) -> (error out=w232:errorcluster)  [unwired: 2 in, 4 out]
              }
              frame False {
              }
            }
          }
          frame "Maximize", "Maximized" {
            w234 = T1."Maximized" ("State")
            n86 = property class="VI"(reference=w240, error in=w239) -> (reference out=w237:refnum<vi>, error out=w238:errorcluster, "FP.State"=w236:T1)
            n87 = Not Equal?(x=w236, y=w234) -> (x != y?=w235:bool)
            n88 = case shown="True" w235 {
              tunnel: [w245 w246] -> w241
              tunnel: w238 -> [w244 w246]
              tunnel: w237 -> [w243 _]
              tunnel: w234 -> [w242 _]
              frame True {
                n89 = invoke class="VI" method="FP.Open"(reference=w243, error in=w244, "State"=w242) -> (error out=w245:errorcluster)  [unwired: 2 in, 4 out]
              }
              frame False {
              }
            }
          }
        }
        n90 = call <vilib>:"Add State(s) to Queue__JKI_lib_State_Machine.vi"("State(s) in (\"\")"=w181) -> ("States Out"=w180:string)  [unwired: 14 in]
      }
      frame "UI: Autoset Arguments" {
        n91 = call "CSM - Revert Arguments-Safe String.vi"("Safe Argument String"=w255) -> ("Origin Argument String"=w247:string)  [unwired: 8 in]
        n92 = control-ref of="CSM"() -> (w250:refnum<vi>)
        n93 = call "Remove Comments from Single-line.vi"("single-line text"=w247) -> ("single-line text without comments"=w254:string)  [unwired: 2 in]
        n94 = call "Split Single-line Message.vi"("single-line text"=w254) -> ("state"=w252:string, "args"=w251:string, "source/target"=w249:string)  [unwired: 6 in, 1 out]
        n95 = case shown="\"<interrupt>\", \"<status>\"" w249 {
          selector: w249 -> [w258 _]
          tunnel: [w258 w259] -> w248
          tunnel: w247 -> [_ w260]
          frame Default {
            (unwired) enum32{"Message", "Status"}."Message" ("Tab(Msg/Status)")
          }
          frame "<interrupt>", "<status>" {
            (unwired) enum32{"Message", "Status"}."Status" ("Tab(Msg/Status)")
            n96 = Match Pattern(string=w260, regular expression="//") -> (after substring=w259:string)  [unwired: 1 in, 3 out]
          }
        }
        n97 = local write "MsgString"(w252) -> ()
        n98 = local write "Arguments"(w251) -> ()
        n99 = property on="Property Node" class="Str"(reference=w250, "Value"=w248) -> ()  [unwired: 1 in, 2 out]
      }
      frame "UI: Refresh History List" {
      }
      frame "CSM: Module Selected" {
        n100 = local write "CSM"(w268) -> ()
        n101 = call <vilib>:"Add State(s) to Queue__jki_lib_state_machine.vi"("State(s) in Front (\"\")"="Action: Refresh API List" ("State(s) in Front (\"\")"), "State(s) in (\"\")"=w266) -> ("States Out"=w267:string)  [unwired: 13 in]
      }
      frame "UI: Refresh UI" {
      }
      frame "UI: Try to Change Command" {
        n102 = call "CSM - Convert HexStr to Data.vi"("HEX String"=w286) -> ("Variant"=w290:variant, "error out"=w291:errorcluster)  [unwired: 7 in]
        n103 = Variant To Data(error in=w291, type="", Variant=w290) -> (data=w288:string)  [unwired: 1 out]
        n104 = call "Remove Comments from Single-line.vi"("single-line text"=w288) -> ("single-line text without comments"=w287:string)  [unwired: 2 in]
        n105 = call "CSM - List Modules.vi"("Scope (Normal)"=_CSM_List_Module_Scope."All") -> ("Module Names"=w282:string[])  [unwired: 9 in, 1 out]
        n106 = call "Split Single-line Message.vi"("single-line text"=w287) -> ("state"=w275:string, "args"=w278:string, "source/target"=w279:string)  [unwired: 6 in, 1 out]
        n107 = To Lower Case(string=w282) -> (all lower case string=w284:string[])
        n108 = To Lower Case(string=w279) -> (all lower case string=w283:string)
        n109 = Search 1D Array(1D array=w284, element=w283) -> (index of element=w281:i32)  [unwired: 1 in]
        n110 = Greater Or Equal To 0?(x=w281) -> (x >= 0?=w280:bool)
        n111 = case shown="True" w280 {
          tunnel: w279 -> [_ w298]
          tunnel: w278 -> [_ w297]
          tunnel: w275 -> [_ w296]
          tunnel: [_ w295] -> w274
          frame False {
          }
          frame True {
            n112 = call <vilib>:"Build State String with Arguments__JKI_lib_State_Machine.vi"("Arguments (\"\")"=w296, "State"="Action: Refresh API List") -> ("State with Arguments"=w295:string)  [unwired: 4 in]
            n113 = local write "Arguments"(w297) -> ()
            n114 = local write "CSM"(w298) -> ()
          }
        }
        n115 = call <vilib>:"Add State(s) to Queue__jki_lib_state_machine.vi"("State(s) in Front (\"\")"=w274, "State(s) in (\"\")"=w276) -> ("States Out"=w277:string)  [unwired: 13 in]
      }
      frame "---------- Macro ----------" {
        n116 = call <vilib>:"Add State(s) to Queue__JKI_lib_State_Machine.vi"("State(s) in (\"\")"=w302) -> ("States Out"=w301:string)  [unwired: 14 in]
      }
      frame "Macro: Initialize" {
        # "Initialization Macro\n(This is called once, when the VI starts)"
        n117 = call <vilib>:"Add State(s) to Queue__JKI_lib_State_Machine.vi"("State(s) in Front (\"\")"="Data: Initialize\nData: Initialize References\nInitialize Core Data\nUI: Initialize\n//UI: Front Panel State >> Open\nAction: Refresh API List\nAction: Change Btn States", "State(s) in (\"\")"=w307) -> ("States Out"=w306:string)  [unwired: 13 in]
      }
      frame "Macro: Exit" {
        # "Exit Macro\n(This is called once, when the VI exits)"
        n118 = call "_Broadcast Message.vi"("Broadcast"=_BroadcastDef."Macro: Exit") -> ()  [unwired: 10 in, 1 out]
        n119 = call <vilib>:"Add State(s) to Queue__JKI_lib_State_Machine.vi"("State(s) at Back (\"\")"="Data: Cleanup\nExit") -> ("States Out"=w309:string)  [unwired: 14 in]
        n120 = call <vilib>:"Add State(s) to Queue__JKI_lib_State_Machine.vi"("State(s) in Front (\"\")"=w309, "State(s) in (\"\")"=w314) -> ("States Out"=w313:string)  [unwired: 13 in]
      }
      frame "---------- Action ----------" {
        # "Template Separator\n(You can make a copy of, or modify, this frame)"
        n121 = call <vilib>:"Add State(s) to Queue__JKI_lib_State_Machine.vi"("State(s) in (\"\")"=w318) -> ("States Out"=w317:string)  [unwired: 14 in]
      }
      frame "Action: Send CSM Message" {
        n122 = local read "CSM"() -> (w322:string)
        n123 = Multiply(x=1000, y="Timeout(s)") -> (x*y=w320:i32)
        n124 = case shown="Default" "MsgString" {
          selector: "MsgString" -> [_ w336]
          tunnel: "Arguments" -> [_ w335]
          tunnel: [_ w338] -> w323
          tunnel: w322 -> [_ w334]
          tunnel: w320 -> [_ w337]
          frame "" {
          }
          frame Default {
            n125 = call "CSM - Send Message and Wait for Reply.vi"("Response Timeout (-2 Using Global Settings)"=w337, "Current Module (\"\" to Generate an ID)"="Tool-Testpnl" ("Current Module(\"\" to generate an ID)"), "Target Module"=w334, "Arguments (\"\")"=w335, "State"=w336) -> ("error out"=w338:errorcluster, "Response"=w340:string)  [unwired: 4 in, 1 out]
            n126 = call-poly "Build Message with Arguments++.vi"("State With Arguments"=w336, "Arguments (\"\")"=w335, "Target Module (\"\")"=w334) -> ("CSM Message String"=w331:string)  [unwired: 12 in]
            n127 = case shown="True" "Revert Safe String" {
              tunnel: w340 -> [w341 w343]
              tunnel: [w341 w342] -> w333
              frame False {
              }
              frame True {
                n128 = call "CSM - Revert Arguments-Safe String.vi"("Safe Argument String"=w343) -> ("Origin Argument String"=w342:string)  [unwired: 8 in]
              }
            }
            "Response" <- w333
            n129 = call "CSM - Convert Data to HexStr.vi"("Variant"=w331) -> ("HEX String (0-9,A-F)"=w330:string)  [unwired: 8 in]
            n130 = call "_Broadcast Message.vi"("Argument(\"\")"=w330, "Broadcast"=_BroadcastDef."CSM: Message Excuted") -> ()  [unwired: 9 in, 1 out]
          }
        }
        n131 = call <vilib>:"Simple Error Handler.vi"("error in (no error)"=w323) -> ()  [unwired: 4 in, 5 out]
        n132 = call <vilib>:"Add State(s) to Queue__JKI_lib_State_Machine.vi"("State(s) in (\"\")"=w328) -> ("States Out"=w327:string)  [unwired: 14 in]
      }
      frame "Action: Post CSM Message" {
        # "Your code here.\n(You can make a copy of, or modify, this frame)"
        n133 = local read "MsgString"() -> (w344:string)
        n134 = local read "Arguments"() -> (w345:string)
        n135 = local read "CSM"() -> (w346:string)
        n136 = case shown="Default" w344 {
          selector: w344 -> [_ w356]
          tunnel: w345 -> [_ w355]
          tunnel: [_ w357] -> w347
          tunnel: w346 -> [_ w354]
          frame "" {
          }
          frame Default {
            (unwired) "CSM: Message Excuted" ("State")
            n137 = call-poly "Build Message with Arguments++.vi"("State With Arguments"=w356, "Arguments (\"\")"=w355, "Target Module (\"\")"=w354) -> ("CSM Message String"=w353:string)  [unwired: 12 in]
            n138 = call "CSM - Post Message.vi"("Current Module (\"\" to Generate an ID)"="Tool-Testpnl" ("Current Module(\"\" to generate an ID)"), "Target Module"=w354, "Arguments (\"\")"=w355, "State"=w356) -> ("error out"=w357:errorcluster)  [unwired: 7 in]
            n139 = call "CSM - Convert Data to HexStr.vi"("Variant"=w353) -> ("HEX String (0-9,A-F)"=w352:string)  [unwired: 8 in]
            n140 = call "_Broadcast Message.vi"("Argument(\"\")"=w352, "Broadcast"=_BroadcastDef."CSM: Message Excuted") -> ()  [unwired: 9 in, 1 out]
          }
        }
        n141 = call <vilib>:"Simple Error Handler.vi"("error in (no error)"=w347) -> ()  [unwired: 4 in, 5 out]
        n142 = call <vilib>:"Add State(s) to Queue__JKI_lib_State_Machine.vi"("State(s) in (\"\")"=w350) -> ("States Out"=w349:string)  [unwired: 14 in]
      }
      frame "Action: Broadcast Status" {
        # "Your code here.\n(You can make a copy of, or modify, this frame)"
        n143 = local read "MsgString"() -> (w359:string)
        n144 = local read "Arguments"() -> (w360:string)
        n145 = local read "CSM"() -> (w362:string)
        n146 = case shown="Default" w359 {
          selector: w359 -> [_ w369]
          tunnel: w360 -> [_ w368]
          tunnel: [_ w370] -> w363
          tunnel: w362 -> [_ w367]
          tunnel: [_ w375] -> w361
          frame "" {
          }
          frame Default {
            (unwired) "Tool-Testpnl" ("Current Module(\"\" to generate an ID)")
            n147 = call "CSM - Request CSM to Broadcast Status Change.vi"("Module Name"=w367, "Arguments (\"\")"=w368, "Status"=w369) -> ("error out"=w370:errorcluster)  [unwired: 8 in]
            n148 = call-poly "Build Message with Arguments++.vi"("State With Arguments"=w369, "Arguments (\"\")"=w368) -> ("CSM Message String"=w377:string)  [unwired: 13 in]
            n149 = Concatenate Strings(w377, "//" ("string"), w367) -> (w372:string)
            n150 = call "CSM - Make String Arguments Safe.vi"("Argument String"=w372) -> ("Safe Argument String"=w376:string)  [unwired: 8 in]
            n151 = call <vilib>:"Build State String with Arguments__JKI_lib_State_Machine.vi"("Arguments (\"\")"=w376, "State"="" ("State(s) in Front (\"\")")) -> ("State with Arguments"=w374:string)  [unwired: 4 in]
            n152 = call <vilib>:"Add State(s) to Queue__JKI_lib_State_Machine.vi"("State(s) in (\"\")"=w374, "State(s) at Back (\"\")"="UI: Refresh History List" ("State(s) in Front (\"\")")) -> ("States Out"=w375:string)  [unwired: 13 in]
          }
        }
        n153 = call <vilib>:"Add State(s) to Queue__JKI_lib_State_Machine.vi"("State(s) in (\"\")"=w366, "State(s) at Back (\"\")"=w361) -> ("States Out"=w365:string)  [unwired: 13 in]
      }
      frame "Action: Change Btn States" {
      }
      frame "Action: Refresh API List" {
        n154 = local read "CSM"() -> (w392:string)
        n155 = call "CSM - Check If Module Exists.vi"("CSM Name"=w392) -> ("error out"=w390:errorcluster, "Exist?"=w388:bool, "CSM Name (Dup)"=w391:string)  [unwired: 8 in]
        n156 = case shown="True" w388 {
          tunnel: w391 -> [_ w406]
          tunnel: w390 -> [_ w405]
          tunnel: w389 -> [_ w402]
          tunnel: [_ w397] -> w385
          frame False {
          }
          frame True {
            n157 = call "CSM - Module VI Reference.vi"("Current Module (\"\" to Generate an ID)"=w402, "error in (no error)"=w405, "CSM Name"=w406) -> ("error out"=w403:errorcluster, "CSM Module VIRef"=w404:refnum<vi>)  [unwired: 7 in]
            n158 = call <vilib>:"Get User VI Tag.vi"("error in (no error)"=w403, "Tag Name"="CSM.PythonWrapper", "VI Refnum"=w404) -> ("error out"=w400:errorcluster, "Value"=w399:variant)  [unwired: 5 in, 2 out]
            n159 = Variant To Data(error in=w400, type=FALSE, Variant=w399) -> (data=w397:bool)  [unwired: 1 out]
          }
        }
        n160 = Select(t="Action: Refresh Python API List", s=w385, f="Action: Refresh LV API List") -> (s? t:f=w383:string)
        n161 = call <vilib>:"Build State String with Arguments__JKI_lib_State_Machine.vi"("Arguments (\"\")"=w382, "State"=w383) -> ("State with Arguments"=w384:string)  [unwired: 4 in]
        n162 = call <vilib>:"Add State(s) to Queue__JKI_lib_State_Machine.vi"("State(s) in Front (\"\")"=w384, "State(s) in (\"\")"=w393) -> ("States Out"=w394:string)  [unwired: 13 in]
      }
      frame "Action: Refresh LV API List" {
        # "argument is selected state"
        n163 = local read "CSM"() -> (w412:string)
        n164 = in-place {
          in-place-border: w412 -> [w422]
          in-place-border: [w421] -> w415
          n165 = in-place-cluster #1(w414) -> ("CSM Check History"=w420:string[])
          n166 = Search 1D Array(1D array=w420, element=w422) -> (index of element=w423:i32)  [unwired: 1 in]
          n167 = Less Than 0?(x=w423) -> (x < 0?=w421:bool)
          n168 = case shown="True" w421 {
            tunnel: w420 -> [w424 w427]
            tunnel: w422 -> [_ w426]
            tunnel: [w424 w425] -> w419
            frame False {
            }
            frame True {
              n169 = Build Array (concatenate)(w427, w426) -> (w425:string[])
            }
          }
          n170 = in-place-cluster #1("CSM Check History"=w419) -> (w413:T6)
        }
        n171 = call "CSM - Check If Module Exists.vi"("CSM Name"=w412) -> ("error out"=w409:errorcluster, "Exist?"=w410:bool, "CSM Name (Dup)"=w417:string)  [unwired: 8 in]
        n172 = Not(x=w409) -> (.not. x?=w408:bool)
        n173 = And(x=w410, y=w408) -> (x .and. y?=w411:bool)
        n174 = case shown="True" w411 {
          tunnel: w417 -> [_ w431]
          tunnel: w416 -> [_ w432]
          tunnel: w415 -> [_ w433]
          tunnel: w407 -> [_ w430]
          frame False {
            w429 = T8."Disabled and Grayed Out" ("Disabled")
            n175 = property on="Message/Status" class="CmbBox"("Strings[]"=string[] [] ("Strings []")) -> ()  [unwired: 2 in, 2 out]
            n176 = property on="Revert Safe String" class="Bool (strict)"("DisabledEnum"=w429) -> ()  [unwired: 2 in, 2 out]
            n177 = property on="Arguments" class="Str"("DisabledEnum"=w429) -> ()  [unwired: 2 in, 2 out]
            n178 = property on="Response" class="Str"("DisabledEnum"=w429) -> ()  [unwired: 2 in, 2 out]
          }
          frame True {
            w436 = T8."Enabled" ("Disabled")
            n179 = control-ref of="MsgString"() -> (w434:refnum<vi>)
            n180 = control-ref of="Interface-Filter"() -> (w435:refnum<vi>)
            n181 = call "_Autofill API CmbBox.vi"("CmbBox"=w434, "Current Module (\"\" to Generate an ID)"=w432, "CSM Name"=w431, "API Name"=w430, "Force? (F)"=w433, "Interface-Filter"=w435) -> ()  [unwired: 9 in, 1 out]
            n182 = property on="Arguments" class="Str"("DisabledEnum"=w436) -> ()  [unwired: 2 in, 2 out]
            n183 = property on="Response" class="Str"("DisabledEnum"=w436) -> ()  [unwired: 2 in, 2 out]
            n184 = property on="Revert Safe String" class="Bool (strict)"("DisabledEnum"=w436) -> ()  [unwired: 2 in, 2 out]
          }
        }
      }
      frame "Action: Refresh Python API List" {
        # "argument is selected state"
        n185 = local read "CSM"() -> (w442:string)
        n186 = in-place {
          in-place-border: w442 -> [w452]
          in-place-border: [w451] -> w445
          n187 = in-place-cluster #2(w444) -> ("CSM Check History"=w450:string[])
          n188 = Search 1D Array(1D array=w450, element=w452) -> (index of element=w453:i32)  [unwired: 1 in]
          n189 = Less Than 0?(x=w453) -> (x < 0?=w451:bool)
          n190 = case shown="True" w451 {
            tunnel: w450 -> [w454 w457]
            tunnel: w452 -> [_ w456]
            tunnel: [w454 w455] -> w449
            frame False {
            }
            frame True {
              n191 = Build Array (concatenate)(w457, w456) -> (w455:string[])
            }
          }
          n192 = in-place-cluster #2("CSM Check History"=w449) -> (w443:T6)
        }
        n193 = call "CSM - Check If Module Exists.vi"("CSM Name"=w442) -> ("error out"=w439:errorcluster, "Exist?"=w440:bool, "CSM Name (Dup)"=w447:string)  [unwired: 8 in]
        n194 = Not(x=w439) -> (.not. x?=w438:bool)
        n195 = And(x=w440, y=w438) -> (x .and. y?=w441:bool)
        n196 = case shown="True" w441 {
          tunnel: w447 -> [_ w462]
          tunnel: w446 -> [_ w478]
          tunnel: w445 -> [_ w480]
          tunnel: w437 -> [_ w460]
          frame False {
            w459 = T8."Disabled and Grayed Out" ("Disabled")
            n197 = property on="Message/Status" class="CmbBox"("Strings[]"=string[] [] ("Strings []")) -> ()  [unwired: 2 in, 2 out]
            n198 = property on="Revert Safe String" class="Bool (strict)"("DisabledEnum"=w459) -> ()  [unwired: 2 in, 2 out]
            n199 = property on="Arguments" class="Str"("DisabledEnum"=w459) -> ()  [unwired: 2 in, 2 out]
            n200 = property on="Response" class="Str"("DisabledEnum"=w459) -> ()  [unwired: 2 in, 2 out]
          }
          frame True {
            w481 = T8."Enabled" ("Disabled")
            n201 = call "Read CSM States with lvcsm Support.vi"("Current Module (\"\" to Generate an ID)"=w478, "Force? (F)"=w480, "CSM Name"=w462) -> ("error out"=w479:errorcluster, "CSMAPI List"=w469:string[])  [unwired: 7 in]
            n202 = local read "Interface-Filter"() -> (w468:enum16{"API-Only", "UserDef States", "All"})
            n203 = call "CSM - Send Message and Wait for Reply.vi"("Current Module (\"\" to Generate an ID)"=w478, "Error In (No Error)"=w479, "Target Module"=w462, "State"="Python: List API") -> ("Response"=w476:string)  [unwired: 5 in, 2 out]
            n204 = control-ref of="MsgString"() -> (w461:refnum<vi>)
            n205 = Match Pattern(string=w476, regular expression="^[\\[]?" ("State")) -> (after substring=w475:string)  [unwired: 1 in, 3 out]
            n206 = Match Pattern(string=w475, regular expression="[\\]]?$" ("State")) -> (before substring=w474:string)  [unwired: 1 in, 3 out]
            n207 = call "String to 1D Array_csm.vi"("delimiter (Tab)"=",", "string"=w474) -> ("Array of Strings"=w470:string[])  [unwired: 9 in]
            n208 = case shown="\"All\"" w468 {
              tunnel: w470 -> [w484 w487]
              tunnel: w469 -> [_ w486]
              tunnel: [w484 w485] -> w465
              frame Default {
              }
              frame "All" {
                n209 = Build Array (concatenate)(w487, w486) -> (w485:string[])
              }
            }
            n210 = for {
              tunnel: w465 -> [w483] mode=indexing
              tunnel: [w482] -> w463 mode=indexing
              n211 = call <vilib>:"Trim Whitespace.vi"("string"=w483) -> ("trimmed string"=w482:string)  [unwired: 1 in]
            }
            n212 = property on="Arguments" class="Str"("DisabledEnum"=w481) -> ()  [unwired: 2 in, 2 out]
            n213 = property on="Response" class="Str"("DisabledEnum"=w481) -> ()  [unwired: 2 in, 2 out]
            n214 = property on="Revert Safe String" class="Bool (strict)"("DisabledEnum"=w481) -> ()  [unwired: 2 in, 2 out]
            n215 = Empty String/Path?(string/path=w460) -> (empty?=w467:bool)
            n216 = Index Array(array=w463) -> (element=w466:string)  [unwired: 1 in]
            n217 = Select(t=w466, s=w467, f=w460) -> (s? t:f=w464:string)
            n218 = property class="CmbBox"(reference=w461, "Strings[]"=w463, "Value"=w464) -> ()  [unwired: 1 in, 2 out]
          }
        }
      }
      frame "No Peroidic Log over 1s" {
      }
    }
  }
  n219 = disable-structure shown="Disabled" {
    frame Disabled {
      n220 = case shown="\"Module Created\", \"Module Destroyed\"" {
        selector: _ -> [_ _]
        tunnel: _ -> [_ w492]
        frame "User Log", Default {
        }
        frame "Module Created", "Module Destroyed" {
          n221 = Generate User Event(user event=w492, event data cluster="UI: Refresh CSM List" ("State(s) in Front (\"\")")) -> ()  [unwired: 2 in, 2 out]
        }
      }
    }
    frame Enabled {
    }
  }
  n222 = control-ref of="Current VI Reference"() -> (w4:refnum<vi>)
  n223 = call "Close FP if in LabVIEW Dir.vi"("VI Refnum"=w4, "Error in"=w3) -> ("Error out"=w5:errorcluster)  [unwired: 9 in]
  n224 = call <vilib>:"Clear Errors.vi"("error in (no error)"=w5) -> ()  [unwired: 5 in, 2 out]
